vi "Display Control Value.vi"(4 "Display Control":T1) -> (7 "DCtrl Value":u8)   [LabVIEW 2020, in "CTI-Peripheral.lvlib" / "HD44780 LCD.lvlib"]
uses:
  HD44780 LCD.lvlib
  Display Control.ctl
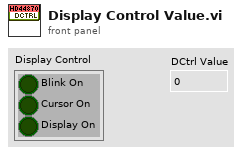
[diagram p1: front panel]
types:
  T1 = typedef "CTI-Peripheral.lvlib/HD44780 LCD.lvlib/Display Control.ctl" = cluster{"Blink On":bool, "Cursor On":bool, "Display On":bool}
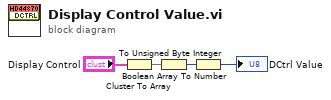
[diagram p0: block diagram]
diagram:
  n1 = Cluster To Array(cluster="Display Control") -> (array=w3:bool[])
  n2 = Boolean Array To Number(Boolean array=w3) -> (number=w2:u32)
  n3 = To Unsigned Byte Integer(number=w2) -> (unsigned 8bit integer=→"DCtrl Value":u8)
